vi "Add To List.vi"(8 "error in (no error)":errorcluster, 10 "Item":string, 11 "StringList Reference":refnum<data-value>) -> (0 "error out":errorcluster, 3 "StringList Reference":refnum<data-value>)   [LabVIEW 2015, in "StringList.lvlib" / "StringList.lvclass"]
uses:
  StringList.lvclass
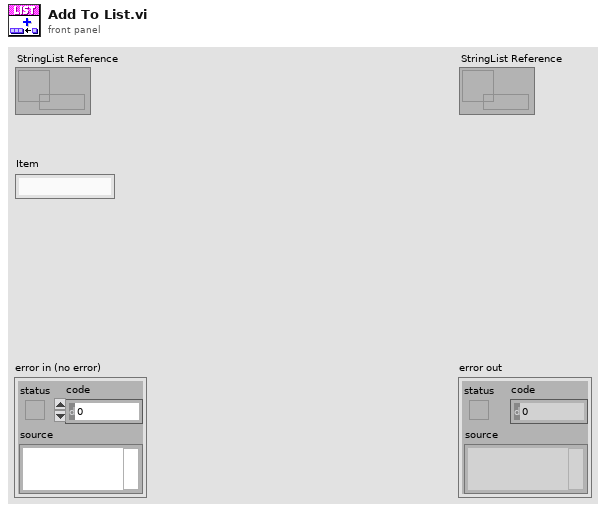
[diagram p1: front panel]
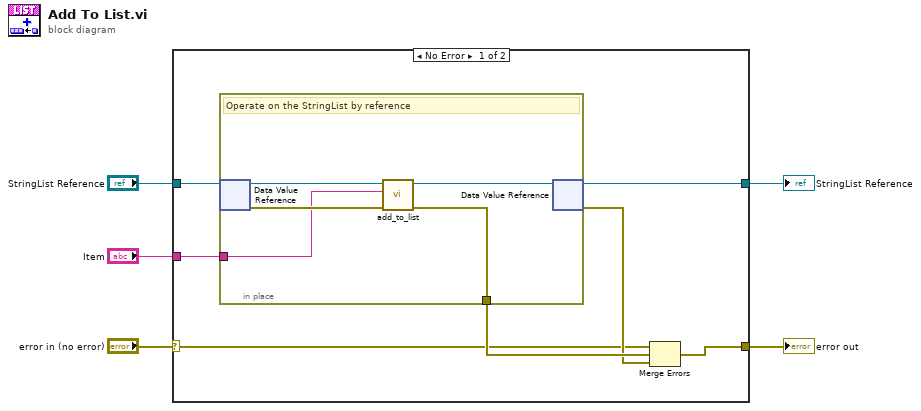
[diagram p0: block diagram]
diagram:
  n1 = case shown="No Error" "error in (no error)" {
    selector: "error in (no error)" -> [w6 w19]
    tunnel: [w12 w19] -> w5
    tunnel: "StringList Reference" -> [w11 w18]
    tunnel: [w10 w18] -> w3
    tunnel: "Item" -> [w9 _]
    frame No Error {
      n2 = in-place {
        in-place-border: w9 -> [w14]
        in-place-border: [w13] -> w8
        # "Operate on the StringList by reference"
        n3 = in-place-dvr #1(w11) -> (w17:refnum<class "StringList.lvclass">, w15:errorcluster)
        n4 = call "add_to_list.vi"("error in (no error)"=w15, "String"=w14, "StringList in"=w17) -> ("error out"=w13:errorcluster, "StringList out"=w16:refnum<class "StringList.lvclass">)  [unwired: 7 in]
        n5 = in-place-dvr #1(w16) -> (w10:refnum<data-value>, w7:errorcluster)
      }
      n6 = Merge Errors(w6, w8, w7) -> (w12:errorcluster)
    }
    frame Error {
    }
  }
  "error out" <- w5
  "StringList Reference" <- w3
